vi "openHelpInDefaultBrowser.vi"(8 "error in (no error)":errorcluster, 11 "name or relative path":string) -> (0 "error out":errorcluster)   [LabVIEW 2017, in "shared.lvlib"]
uses:
  shared.lvlib
  <vilib>/Platform/browser.llb/Open URL in Default Browser (string).vi
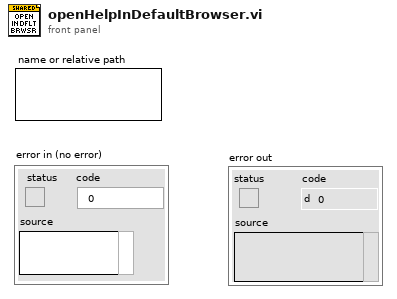
[diagram p1: front panel]
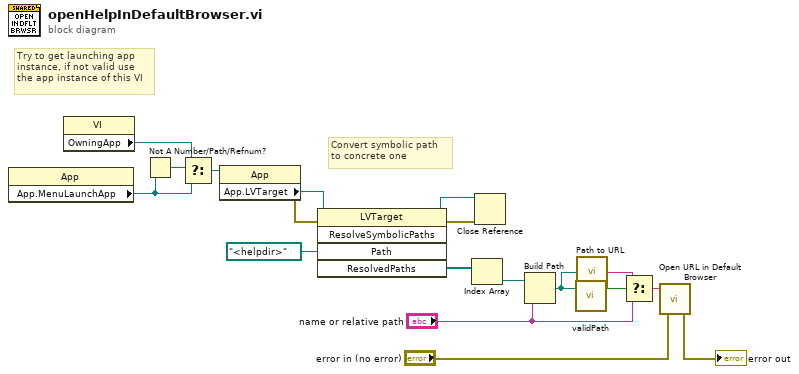
[diagram p0: block diagram]
diagram:
  # "Convert symbolic path\nto concrete one"
  # "Try to get launching app\ninstance, if not valid use\nthe app instance of this VI"
  n1 = property class="App"() -> ("App.MenuLaunchApp"=w8:refnum<vi>)  [unwired: 2 in, 2 out]
  n2 = property class="VI"() -> ("OwningApp"=w9:refnum<vi>)  [unwired: 2 in, 2 out]
  n3 = Not A Number/Path/Refnum?(number/path/refnum=w8) -> (NaN/Path/Refnum?=w10:bool)
  n4 = Select(t=w9, s=w10, f=w8) -> (s? t:f=w7:refnum<vi>)
  n5 = property class="App"(reference=w7) -> (error out=w15:errorcluster, "App.LVTarget"=w14:refnum<vi>)  [unwired: 1 in, 1 out]
  n6 = invoke class="LVTarget" method="ResolveSymbolicPaths"(reference=w14, error in=w15, "Path"=path "<helpdir>" ("base path")) -> (reference out=w11:refnum<vi>, error out=w12:errorcluster, "ResolvedPaths"=w16:path[])  [unwired: 2 in, 2 out]
  n7 = Index Array(array=w16) -> (element=w6:path)  [unwired: 1 in]
  n8 = Close Reference(reference=w11, error in (no error)=w12) -> ()  [unwired: 1 out]
  n9 = Build Path(base path=w6, name or relative path="name or relative path") -> (appended path=w4:path)
  n10 = call "validPath.vi"("Path"=w4) -> ("Valid?"=w3:bool)  [unwired: 18 in]
  n11 = call <vilib>:"Path to URL.vi"("path"=w4) -> ("url"=w2:string)
  n12 = Select(t=w2, s=w3, f="name or relative path") -> (s? t:f=w5:string)
  n13 = call-poly <vilib>:"Open URL in Default Browser.vi"("error in (no error)"="error in (no error)", "URL"=w5) -> ("error out"=→"error out":errorcluster)  [unwired: 4 in, 1 out]
